vi "例5.3“索引数组”函数.vi"() -> ()   [LabVIEW 2017]
panel:
  out "元素":i32
  out "子数组":i32[](array[numeric])
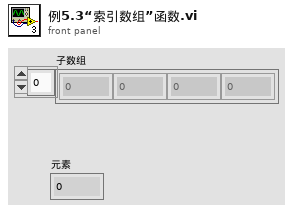
[diagram p1: front panel]
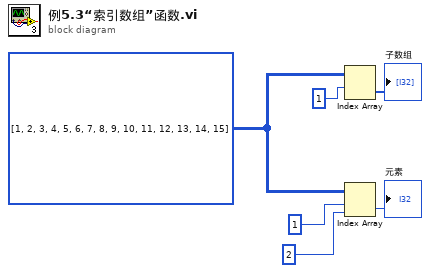
[diagram p0: block diagram]
diagram:
  w4 = i32[][] [[1, 2, 3], [4, 5, 6], [7, 8, 9], [10, 11, 12], [13, 14, 15]]
  n1 = Index Array(array=w4, index (row)=1 ("索引 (行)")) -> (element=→"子数组":i32[])  [unwired: 1 in]
  n2 = Index Array(array=w4, index (row)=1 ("禁用的索引 (行)"), index (col)=2 ("禁用的索引 (列)")) -> (element=→"元素":i32)
